vi "Filtering.vi"(7 "dwelling pixels":i32, 11 "数组输入":dbl[](array[numeric])) -> (3 "数组输出":dbl[](array[numeric]))   [LabVIEW 2013]
uses:
  <vilib>/Analysis/baseanly.llb/Mean (DBL).vi
  <vilib>/Analysis/NI_AALBase.lvlib
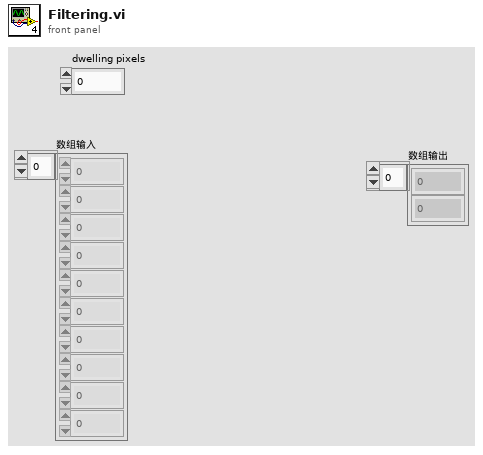
[diagram p1: front panel]
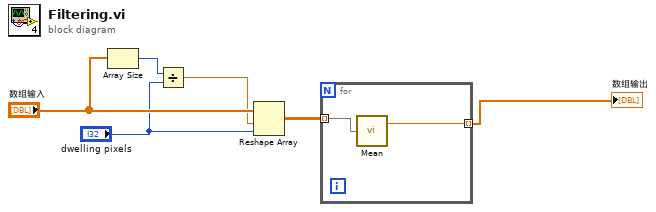
[diagram p0: block diagram]
diagram:
  n1 = Array Size(array="数组输入") -> (size(s)=w5:i32)
  n2 = Divide(x=w5, y="dwelling pixels") -> (x/y=w4:dbl)
  n3 = Reshape Array("数组输入", w4, "dwelling pixels") -> (w2:dbl[][])
  n4 = for {
    tunnel: w2 -> [w8] mode=indexing
    tunnel: [w7] -> w1 mode=indexing
    n5 = call-poly <vilib>:"Mean.vi"("X"=w8) -> ("mean"=w7:dbl)  [unwired: 1 out]
  }
  "数组输出" <- w1
